vi "Pusher_Client_Utility_ErrorHandler.vi"(8 "ErrIn":errorcluster, 10 "Additional Message":string, 11 "Code":i32=-42) -> (0 "ErrOut":errorcluster)   [LabVIEW 2009, in "Client.lvclass"]
uses:
  Client.lvclass
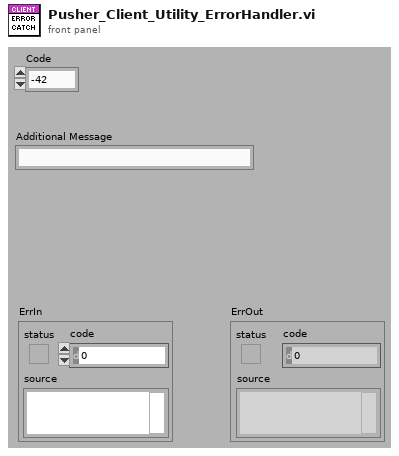
[diagram p1: front panel]
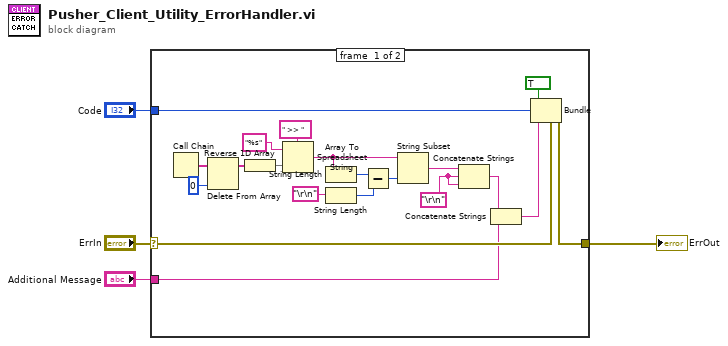
[diagram p0: block diagram]
diagram:
  n1 = case shown="No Error" "ErrIn" {
    selector: "ErrIn" -> [w8 w25]
    tunnel: [w7 w25] -> w3
    tunnel: "Additional Message" -> [w6 _]
    tunnel: "Code" -> [w5 _]
    frame #0 {
      w24 = "\r\n"
      n2 = Call Chain() -> (call chain=w15:string[])
      n3 = Delete From Array(array=w15, index=0 ("Index")) -> (array with subset deleted=w20:string[])  [unwired: 1 in, 1 out]
      n4 = Reverse 1D Array(array=w20) -> (reversed array=w18:string[])
      n5 = Array To Spreadsheet String(delimiter (Tab)=" >> ", array=w18, 3:"%s" ("format string")) -> (spreadsheet string=w21:string)
      n6 = String Length(string=w21) -> (length=w17:i32)
      n7 = String Length(string="\r\n") -> (length=w23:i32)
      n8 = Subtract(x=w17, y=w23) -> (x-y=w16:i32)
      n9 = String Subset(string=w21, length (rest)=w16) -> (substring=w12:string)  [unwired: 1 in]
      n10 = Concatenate Strings(w12, w24, w24) -> (w11:string)
      n11 = Concatenate Strings(w11, w6) -> (w10:string)
      n12 = Bundle(cluster=w8, "status"=TRUE, "code"=w5, "source"=w10) -> (w7:errorcluster)
    }
    frame #1 {
    }
  }
  "ErrOut" <- w3
